vi "RS_gen_command.vi"(3 "error in (no error)":errorcluster, 4 "Comand":string, 5 "address":string="192.168.0.7") -> (0 "error out":errorcluster)   [LabVIEW 2013]
panel:
  # "LIST:SEL '/var/plist1'\nLIST:POW 0dBm, 2dBm, 3dBm\nLIST:RES"
  # "SOUR:LIST:SEL '/hdd/testlist'\n for Linux-based instruments.\n'D:\\testlist'\n for Windows-based instruments.\n SOUR:LIST:FREQ 2 GHz, 4 GHz, 6 GHz, ...\nSOUR:LIST:POW 0 dBm, -10 dBm, 10 dBm, ...\nSOUR:LIST:DWEL 3 ms\nSOUR:LIST:MODE AUTO\nSOUR:LIST:TRIG:SOUR AUTO\nOUTP ON\n*OPC?\nSOUR:LIST:LEAR\n*OPC?\nSOUR:FREQ:MODE LIST"
  # "SOUR:LIST:MODE STEP\nLIST:SEL '/var/plist1'\nCORR:CSET:DATA:FREQ 100MHz,102MHz,103MHz\nCORR:CSET:DATA:POW 1dB, 0.8dB, 0.75dB"
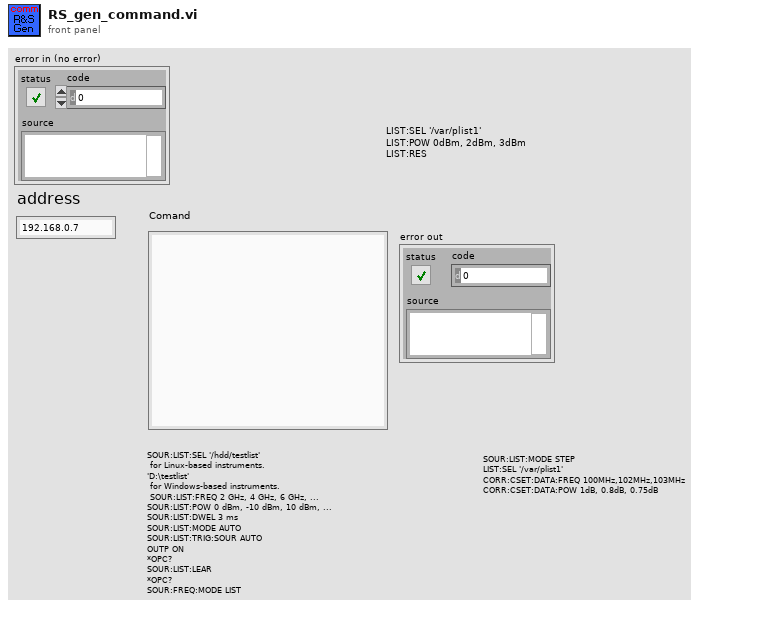
[diagram p1: front panel]
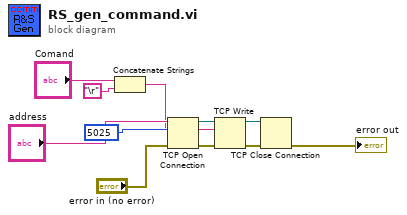
[diagram p0: block diagram]
diagram:
  n1 = Concatenate Strings("Comand", "\r") -> (w2:string)
  n2 = TCP Open Connection(address="address", remote port or service name=u16 5025, error in (no error)="error in (no error)") -> (connection ID=w11:refnum<k5>, error out=w9:errorcluster)  [unwired: 2 in]
  n3 = TCP Write(connection ID=w11, data in=w2, error in (no error)=w9) -> (connection ID out=w10:refnum<k5>, error out=w8:errorcluster)  [unwired: 1 in, 1 out]
  n4 = TCP Close Connection(connection ID=w10, error in (no error)=w8) -> (error out=→"error out":errorcluster)  [unwired: 1 in, 1 out]
